vi "SelectPistonCommand.vi"(1 "Solenoid Selector":T1(ring), 2 "Solenoid Selector State":bool) -> (0 "New State":bool)   [LabVIEW 2020]
uses:
  GlobalDriverStationCommands.vi
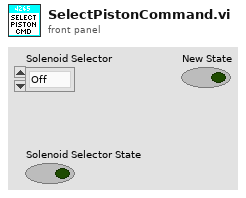
[diagram p1: front panel]
types:
  T1 = enum16{"Off", "Toggle", "D_LT", "D_RT", "D_LB", "D_RB", "D_Y", "D_X", "D_A", "D_B", "M_LT", "M_RT", "M_LB", "M_RB", "M_Y", "M_X", "M_A", "M_B"}
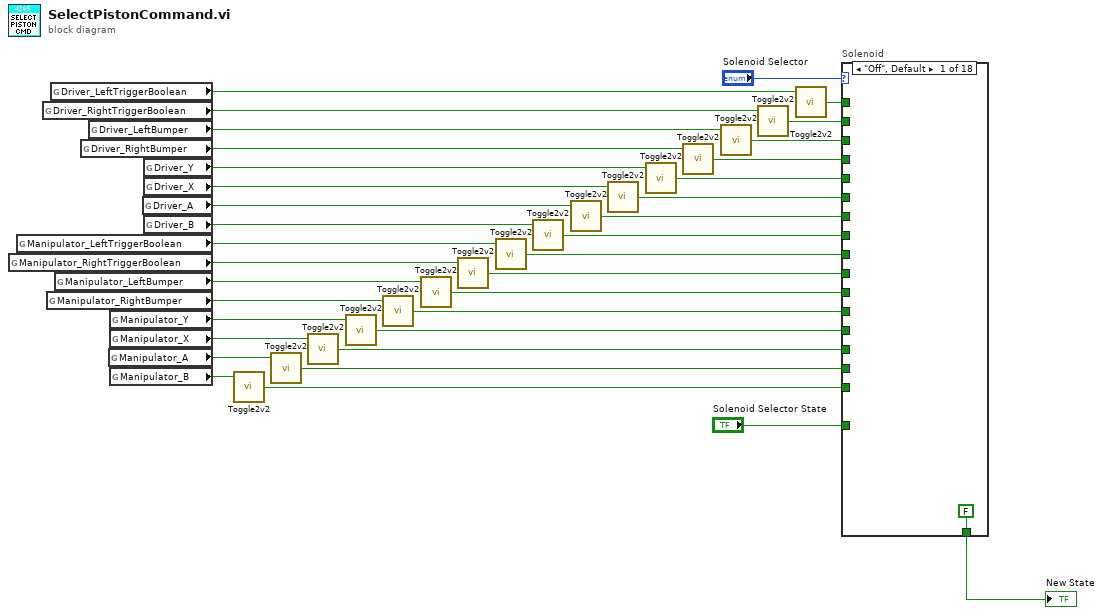
[diagram p0: block diagram]
diagram:
  n1 = global read "GlobalDriverStationCommands.vi" "Manipulator_RightTriggerBoolean"() -> (w23:bool)
  n2 = global read "GlobalDriverStationCommands.vi" "Manipulator_LeftTriggerBoolean"() -> (w21:bool)
  n3 = global read "GlobalDriverStationCommands.vi" "Driver_RightTriggerBoolean"() -> (w6:bool)
  n4 = global read "GlobalDriverStationCommands.vi" "Manipulator_RightBumper"() -> (w27:bool)
  n5 = global read "GlobalDriverStationCommands.vi" "Driver_LeftTriggerBoolean"() -> (w4:bool)
  n6 = global read "GlobalDriverStationCommands.vi" "Manipulator_LeftBumper"() -> (w25:bool)
  n7 = global read "GlobalDriverStationCommands.vi" "Driver_RightBumper"() -> (w11:bool)
  n8 = global read "GlobalDriverStationCommands.vi" "Driver_LeftBumper"() -> (w9:bool)
  n9 = global read "GlobalDriverStationCommands.vi" "Manipulator_A"() -> (w32:bool)
  n10 = global read "GlobalDriverStationCommands.vi" "Manipulator_Y"() -> (w29:bool)
  n11 = global read "GlobalDriverStationCommands.vi" "Manipulator_X"() -> (w30:bool)
  n12 = global read "GlobalDriverStationCommands.vi" "Manipulator_B"() -> (w34:bool)
  n13 = global read "GlobalDriverStationCommands.vi" "Driver_A"() -> (w17:bool)
  n14 = global read "GlobalDriverStationCommands.vi" "Driver_Y"() -> (w13:bool)
  n15 = global read "GlobalDriverStationCommands.vi" "Driver_X"() -> (w14:bool)
  n16 = global read "GlobalDriverStationCommands.vi" "Driver_B"() -> (w18:bool)
  n17 = call "Toggle2v2.vi"("Trigger"=w34) -> ("New State"=w35:bool)  [unwired: 2 in]
  n18 = call "Toggle2v2.vi"("Trigger"=w32) -> ("New State"=w33:bool)  [unwired: 2 in]
  n19 = call "Toggle2v2.vi"("Trigger"=w30) -> ("New State"=w31:bool)  [unwired: 2 in]
  n20 = call "Toggle2v2.vi"("Trigger"=w29) -> ("New State"=w28:bool)  [unwired: 2 in]
  n21 = call "Toggle2v2.vi"("Trigger"=w27) -> ("New State"=w26:bool)  [unwired: 2 in]
  n22 = call "Toggle2v2.vi"("Trigger"=w25) -> ("New State"=w24:bool)  [unwired: 2 in]
  n23 = call "Toggle2v2.vi"("Trigger"=w23) -> ("New State"=w22:bool)  [unwired: 2 in]
  n24 = call "Toggle2v2.vi"("Trigger"=w21) -> ("New State"=w20:bool)  [unwired: 2 in]
  n25 = call "Toggle2v2.vi"("Trigger"=w18) -> ("New State"=w19:bool)  [unwired: 2 in]
  n26 = call "Toggle2v2.vi"("Trigger"=w17) -> ("New State"=w16:bool)  [unwired: 2 in]
  n27 = call "Toggle2v2.vi"("Trigger"=w14) -> ("New State"=w15:bool)  [unwired: 2 in]
  n28 = call "Toggle2v2.vi"("Trigger"=w13) -> ("New State"=w12:bool)  [unwired: 2 in]
  n29 = call "Toggle2v2.vi"("Trigger"=w11) -> ("New State"=w10:bool)  [unwired: 2 in]
  n30 = call "Toggle2v2.vi"("Trigger"=w9) -> ("New State"=w8:bool)  [unwired: 2 in]
  n31 = call "Toggle2v2.vi"("Trigger"=w6) -> ("New State"=w7:bool)  [unwired: 2 in]
  n32 = call "Toggle2v2.vi"("Trigger"=w4) -> ("New State"=w5:bool)  [unwired: 2 in]
  n33 = case "Solenoid" shown="\"Off\", Default" "Solenoid Selector" {
    tunnel: [FALSE ("Manipulator_B") w37 w38 w39 w40 w41 w42 w43 w44 w45 w46 w47 w48 w49 w50 w51 w52 w53] -> w3
    tunnel: "Solenoid Selector State" -> [_ w37 _ _ _ _ _ _ _ _ _ _ _ _ _ _ _ _]
    tunnel: w5 -> [_ _ w38 _ _ _ _ _ _ _ _ _ _ _ _ _ _ _]
    tunnel: w7 -> [_ _ _ w39 _ _ _ _ _ _ _ _ _ _ _ _ _ _]
    tunnel: w8 -> [_ _ _ _ w40 _ _ _ _ _ _ _ _ _ _ _ _ _]
    tunnel: w10 -> [_ _ _ _ _ w41 _ _ _ _ _ _ _ _ _ _ _ _]
    tunnel: w12 -> [_ _ _ _ _ _ w42 _ _ _ _ _ _ _ _ _ _ _]
    tunnel: w15 -> [_ _ _ _ _ _ _ w43 _ _ _ _ _ _ _ _ _ _]
    tunnel: w16 -> [_ _ _ _ _ _ _ _ w44 _ _ _ _ _ _ _ _ _]
    tunnel: w19 -> [_ _ _ _ _ _ _ _ _ w45 _ _ _ _ _ _ _ _]
    tunnel: w20 -> [_ _ _ _ _ _ _ _ _ _ w46 _ _ _ _ _ _ _]
    tunnel: w22 -> [_ _ _ _ _ _ _ _ _ _ _ w47 _ _ _ _ _ _]
    tunnel: w24 -> [_ _ _ _ _ _ _ _ _ _ _ _ w48 _ _ _ _ _]
    tunnel: w26 -> [_ _ _ _ _ _ _ _ _ _ _ _ _ w49 _ _ _ _]
    tunnel: w28 -> [_ _ _ _ _ _ _ _ _ _ _ _ _ _ w50 _ _ _]
    tunnel: w31 -> [_ _ _ _ _ _ _ _ _ _ _ _ _ _ _ w51 _ _]
    tunnel: w33 -> [_ _ _ _ _ _ _ _ _ _ _ _ _ _ _ _ w52 _]
    tunnel: w35 -> [_ _ _ _ _ _ _ _ _ _ _ _ _ _ _ _ _ w53]
    frame "Off", Default {
    }
    frame "Toggle" {
    }
    frame "D_LT" {
    }
    frame "D_RT" {
    }
    frame "D_LB" {
    }
    frame "D_RB" {
    }
    frame "D_Y" {
    }
    frame "D_X" {
    }
    frame "D_A" {
    }
    frame "D_B" {
    }
    frame "M_LT" {
    }
    frame "M_RT" {
    }
    frame "M_LB" {
    }
    frame "M_RB" {
    }
    frame "M_Y" {
    }
    frame "M_X" {
    }
    frame "M_A" {
    }
    frame "M_B" {
    }
  }
  "New State" <- w3
